vi "Write Function.vi"(8 "error in (no error)":errorcluster, 10 "Functions.lvlib:FunctionBase.lvclass":refnum<class "FunctionBase.lvclass">, 11 "Sim_Ideal_PMU in":refnum<class "Sim_Ideal_PMU.lvclass">) -> (0 "error out":errorcluster, 3 "Sim_Ideal_PMU out":refnum<class "Sim_Ideal_PMU.lvclass">)   [LabVIEW 2018, in "SensorPlugins.lvlib" / "Sim_Ideal_PMU.lvclass"]
uses:
  Sim_Ideal_PMU.lvclass
  FGen/MemberClasses/FunctionBaseClass/FunctionBase.lvclass
  Sim_Ideal_PMU.lvclass/Sim_Ideal_PMU.ctl
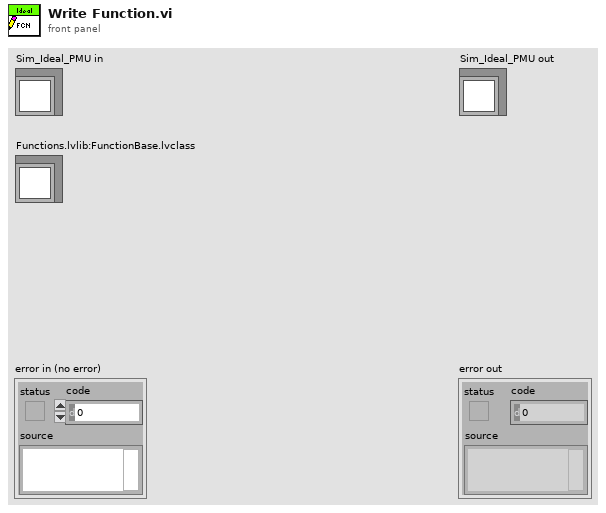
[diagram p1: front panel]
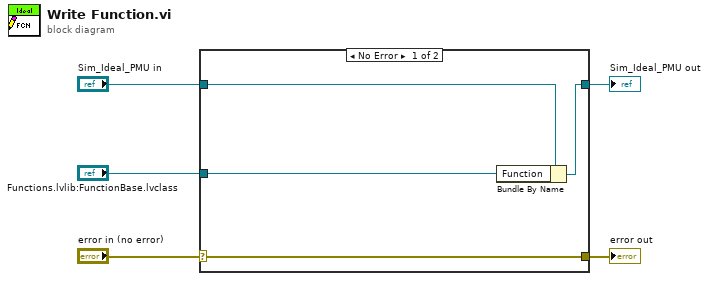
[diagram p0: block diagram]
diagram:
  n1 = case shown="No Error" "error in (no error)" {
    selector: "error in (no error)" -> [w9 w10]
    tunnel: [w9 w10] -> w4
    tunnel: [w7 w11] -> w2
    tunnel: "Sim_Ideal_PMU in" -> [w8 w11]
    tunnel: "Functions.lvlib:FunctionBase.lvclass" -> [w6 _]
    frame No Error {
      n2 = Bundle By Name(cluster=w8, "Function"=w6) -> (w7:refnum<class "Sim_Ideal_PMU.lvclass">)
    }
    frame Error {
    }
  }
  "error out" <- w4
  "Sim_Ideal_PMU out" <- w2
